vi "StopAqcuisition.vi"(8 "error in":errorcluster, 11 "scope in":T1={"scope mode"=enum."Stopped", "ticker"=refnum, "5160 samples per trigger"=0, "FPGA ref"=refnum, "P2P params"={"instrument handle"="", "stream session"=refnum, "scale"={"offset"=0.0, "gain"=0.0, "reserved 1"=0.0, "reserved 2"=0.0}, "actual sample rate"=10000000.0, "Trigger"=enum."PFI 0", "SCOPE Resource"="Dev1", "input impedance"=0}, "data mode"=enum."Real IO", "5782 samples per record"=0, "Chart length"=0} {"P2P params"."input impedance" items=["1 mega ohm"=0, "50 ohms"=2]; "P2P params"."actual sample rate" format="%.2p"}) -> (0 "error out":errorcluster, 3 "scope out":T1={"scope mode"=enum."Stopped", "ticker"=refnum, "5160 samples per trigger"=0, "FPGA ref"=refnum, "P2P params"={"instrument handle"="", "stream session"=refnum, "scale"={"offset"=0.0, "gain"=0.0, "reserved 1"=0.0, "reserved 2"=0.0}, "actual sample rate"=10000000.0, "Trigger"=enum."PFI 0", "SCOPE Resource"="Dev1", "input impedance"=0}, "data mode"=enum."Real IO", "5782 samples per record"=0, "Chart length"=0} {"P2P params"."input impedance" items=["1 mega ohm"=0, "50 ohms"=2]; "P2P params"."actual sample rate" format="%.2p"})   [LabVIEW 2013]
uses:
  controls/scope_params.ctl
  Utilities/Ticker/Ticker.lvclass
  controls/ScopeMode.ctl
  Config/FPGAref.ctl
  P2P streaming/P2P params.ctl
  P2P streaming/trigger_source.ctl
  FPGA/DataMode.ctl
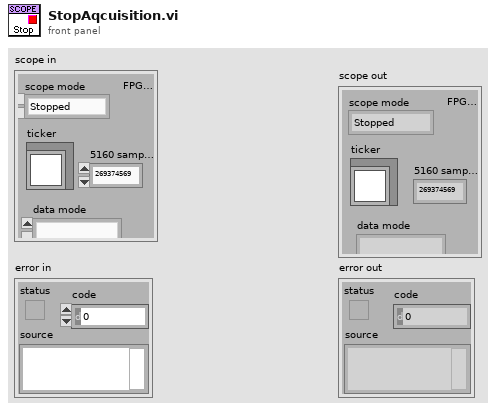
[diagram p1: front panel]
types:
  T1 = typedef "scope_params.ctl" = cluster{"scope mode":T2, "ticker":refnum<class "Ticker.lvclass">, "5160 samples per trigger":u32, "FPGA ref":T3, "P2P params":T4, "data mode":T6, "5782 samples per record":u32, "Chart length":i32}
  T2 = typedef "ScopeMode.ctl" = enum16{"Stopped", "Single", "Running", "Continuous"}
  T3 = typedef "FPGAref.ctl" = refnum<k20>
  T4 = typedef "P2P params.ctl" = cluster{"instrument handle":refnum<k15>, "stream session":refnum<k20>, "scale":cluster{"offset":dbl, "gain":dbl, "reserved 1":dbl, "reserved 2":dbl}, "actual sample rate":dbl, "Trigger":T5, "SCOPE Resource":refnum<k15>, "input impedance":u32}
  T5 = typedef "trigger_source.ctl" = enum16{"PFI 0", "PFI 1", "Software"}
  T6 = typedef "DataMode.ctl" = enum16{"Real IO", "Simulated"}
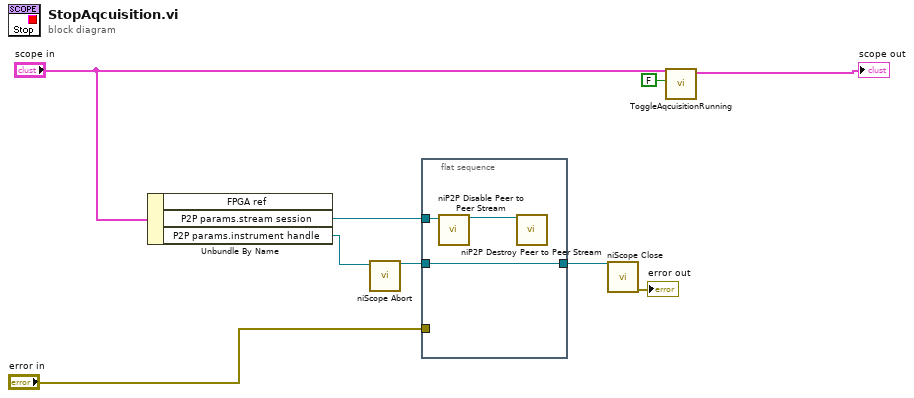
[diagram p0: block diagram]
diagram:
  n1 = Unbundle By Name("scope in") -> ("P2P params.stream session"=w9:refnum<k20>, "P2P params.instrument handle"=w8:refnum<k15>)  [unwired: 1 out]
  n2 = call <instrlib>:"niScope Abort.vi"("instrument handle"=w8) -> ("instrument handle out"=w7:refnum<k15>)  [unwired: 13 in, 1 out]
  n3 = flat-sequence {
    tunnel: w9 -> [w12]
    tunnel: w7 -> [w10]
    tunnel: [w10] -> w6
    tunnel: "error in" -> [_]
    frame #0 {
      n4 = call <vilib>:"niP2P Disable Peer to Peer Stream.vi"("stream session"=w12) -> ("stream session out"=w11:refnum<k20>)  [unwired: 13 in, 1 out]
      n5 = call <vilib>:"niP2P Destroy Peer to Peer Stream.vi"("stream session"=w11) -> ()  [unwired: 14 in, 1 out]
    }
  }
  n6 = call <instrlib>:"niScope Close.vi"("instrument handle"=w6) -> ("error out"=→"error out":errorcluster)  [unwired: 14 in]
  n7 = call "ToggleAqcuisitionRunning.vi"("Acquisition running"=FALSE, "scope in"="scope in") -> ("scope out"=→"scope out":T1)  [unwired: 8 in, 1 out]
